vi "Get Queue Encode.vi"(8 "error in (no error)":errorcluster) -> (0 "error out":errorcluster, 3 "Decoder Queue":refnum<queue>)   [LabVIEW 2023, in "Encoder.lvlib"]
uses:
  Encoder.lvlib
  Internal Communication/Controls/State FGV.ctl
  Internal Communication/Internal Communication.lvlib
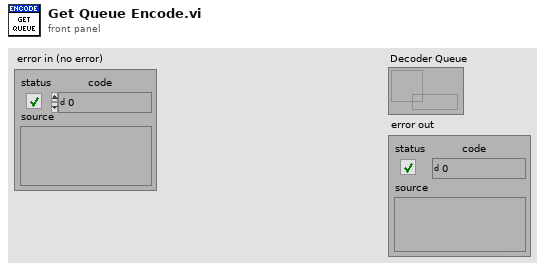
[diagram p1: front panel]
types:
  T1 = typedef "Internal Communication.lvlib/State FGV.ctl" = enum16{"Create Queues", "Get Queues", "Destroy Queues"}
  T2 = typedef "Internal Communication.lvlib/Queues Control.ctl" = cluster{"Heart":refnum<queue>, "FPGA":refnum<queue>, "Encoder":refnum<queue>, "Decoder":refnum<queue>, "Error":refnum<queue>, "UI":refnum<queue>}
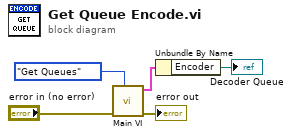
[diagram p0: block diagram]
diagram:
  n1 = call "Main VI.vi"("Enum"=State_FGV."Get Queues", "error in (no error)"="error in (no error)") -> ("error out"=→"error out":errorcluster, "Queues"=w5:T2)  [unwired: 8 in]
  n2 = Unbundle By Name(w5) -> ("Encoder"=→"Decoder Queue":refnum<queue>)
